vi "SVR.vi"(0 "System no.":i32=1 min=1 max=4 step=1, 2 "Axes to move":string[](array[string]), 3 "PZT voltage":dbl[](array[numeric]) format="%.6f", 4 "No.of digits":i16=4, 5 "error in":errorcluster) -> (19 "error out":errorcluster)   [LabVIEW 2020]
doc: "Sets relative PZT voltage for specified axes. Servo must be switched off (using SVO.vi) before using this command. No. of digits is the number of digits after the decimal point in the voltage value(s) that will be sent.\n\nE-517, E-518: Motion commands like SVR are not allowed when the controller is in OFFLINE mode or when the wave generator output is active. When a macro is running on the controller, SVR will be executed not until the macro is finished or stopped. See \"Control Value Generation\" and \"Control Modes\" in the controller user manual for details.\n\nC-413, E-709: Motion commands are not allowed when a wave generator is active or the analog input is used for target generation.\n\nE-712: SVR is valid for axes driven by conventional piezo actuators only. PZT voltage is a dimensionsless value whose range corresponds approximately to the mechanics travel range in µm. Motion commands are not allowed when a wave generator is active or the analog input is used for target generation.\n\nE-725, E-727: PZT voltage is a dimensionsless value whose range corresponds approximately to the mechanics travel range in µm. Motion commands are not allowed when a wave generator is active or the analog input is used for target generation.\n\nE-753, E-754: PZT voltage is a dimensionsless value whose range corresponds approximately to the mechanics travel range in µm. Motion commands are not allowed when the wave generator is active or the analog input is used for target generation.\n\nE-761: PZT voltage is a dimensionsless value whose range corresponds approximately to the mechanics travel range in µm. Motion commands are not allowed when a wave generator is active.\n\nE-816: Only one axis per command allowed. It is necessary to wait a certain time before sending the next command to prevent it from being lost."
panel:
  # "Sets relative PZT voltage for specified axes."
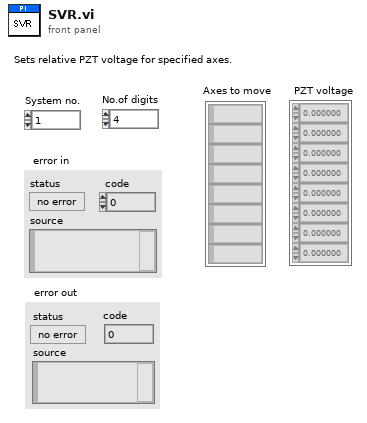
[diagram p1: front panel]
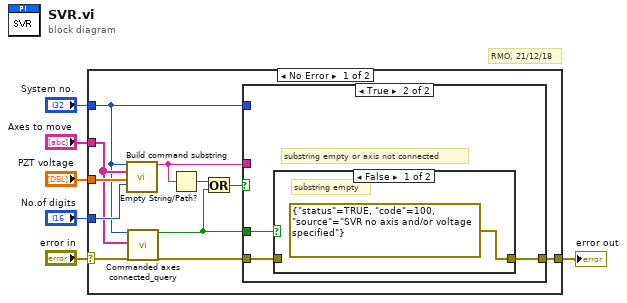
[diagram p0: block diagram]
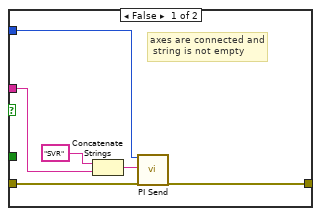
[diagram p2: hidden frame]
diagram:
  # "RMO, 21/12/18"
  n1 = case shown="No Error" "error in" {
    selector: "error in" -> [w11 w29]
    tunnel: [w17 w29] -> w6
    tunnel: "PZT voltage" -> [w16 _]
    tunnel: "No.of digits" -> [w15 _]
    tunnel: "System no." -> [w12 _]
    tunnel: "Axes to move" -> [w13 _]
    frame No Error {
      n2 = call "Build command substring.vi"("System no."=w12, "Affected axes"=w13, "Parameters"=w16, "No. of digits"=w15) -> ("Command substring"=w10:string)  [unwired: 3 in, 12 out]
      n3 = call "Commanded axes connected_query.vi"("System no."=w12, "Commanded axes"=w13, "error in"=w11) -> ("Controller error"=w8:bool, "error out"=w14:errorcluster)  [unwired: 1 in, 14 out]
      n4 = Empty String/Path?(string/path=w10) -> (empty?=w9:bool)
      n5 = Or(x=w9, y=w8) -> (x .or. y?=w7:bool)
      n6 = case shown="True" w7 {
        tunnel: w10 -> [w22 _]
        tunnel: [w19 w26] -> w17
        tunnel: w14 -> [w20 w24]
        tunnel: w8 -> [_ w25]
        tunnel: w12 -> [w18 _]
        frame False {
          # "axes are connected and\n string is not empty"
          n7 = Concatenate Strings("SVR", w22) -> (w21:string)
          n8 = call "PI Send.vi"("System no."=w18, "String to send"=w21, "error in"=w20) -> ("error out"=w19:errorcluster)  [unwired: 3 in, 13 out]
        }
        frame True {
          # "substring empty or axis not connected"
          n9 = case shown="False" w25 {
            tunnel: [errorcluster {"status"=TRUE, "code"=100, "source"="SVR no axis and/or voltage specified"} ("error out") w28] -> w26
            tunnel: w24 -> [_ w28]
            frame False {
              # "substring empty"
            }
            frame True {
              # "commanded axis not connected"
            }
          }
        }
      }
    }
    frame Error {
    }
  }
  "error out" <- w6
